vi "toCompiledXml.vi"(8 "error in (no error)":errorcluster, 11 "ScriptEvent in":refnum<class "ScriptEvent.lvclass">) -> (0 "error out":errorcluster, 2 "compiledXML":refnum<class "xmlNode.lvclass">, 3 "ScriptEvent out":refnum<class "ScriptEvent.lvclass">)   [LabVIEW 2011, in "Tools.lvlib" / "Scripting.lvlib" / "ScriptEvent.lvclass"]
uses:
  ScriptEvent.lvclass
  xmlNode/xmlNode.lvclass
  ScriptEvent.lvclass/ScriptEvent.ctl
  DatabaseHelpers/Database Objects/Channel/Channel.lvclass
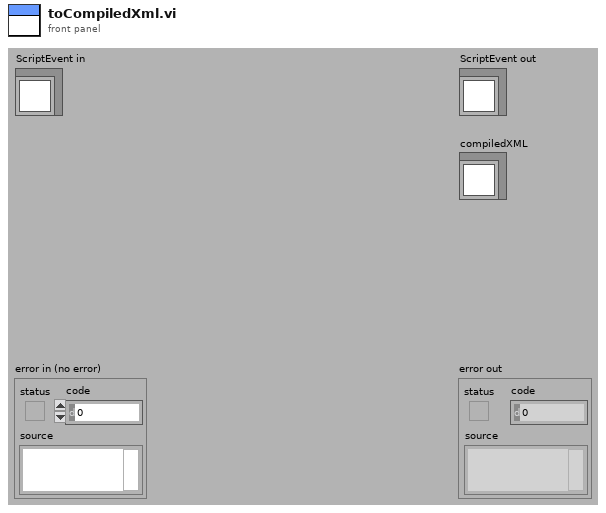
[diagram p1: front panel]
types:
  T1 = cluster{"attributeName":string, "channel_name":string}
  T2 = cluster{"attributeName":string, "channel_name":string}[]
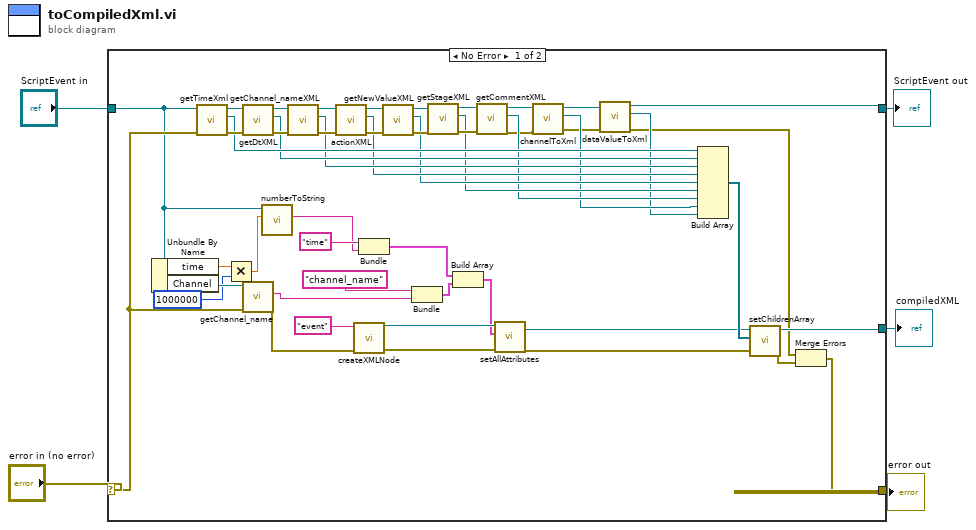
[diagram p0: block diagram]
diagram:
  n1 = case shown="No Error" "error in (no error)" {
    selector: "error in (no error)" -> [w40 w57]
    tunnel: [w29 w57] -> w2
    tunnel: [w7 w56] -> w4
    tunnel: "ScriptEvent in" -> [w14 w56]
    tunnel: [w31 _] -> w1
    frame No Error {
      n2 = Unbundle By Name(w14) -> ("time"=w18:dbl, "Channel"=w54:refnum<class "Channel.lvclass">)
      n3 = call "getTimeXml.vi"("error in (no error)"=w40, "ScriptEvent in"=w14) -> ("error out"=w52:errorcluster, "timeXML"=w39:refnum<class "xmlNode.lvclass">, "ScriptEvent out"=w46:refnum<class "ScriptEvent.lvclass">)  [unwired: 7 in]
      n4 = Multiply(x=w18, y=1000000) -> (x*y=w16:dbl)
      n5 = call "getDtXML.vi"("error in (no error)"=w52, "ScriptEvent in"=w46) -> ("error out"=w51:errorcluster, "dtXML"=w38:refnum<class "xmlNode.lvclass">, "ScriptEvent out"=w45:refnum<class "ScriptEvent.lvclass">)  [unwired: 7 in]
      n6 = call "getChannel_name.vi"("error in (no error)"=w40, "Channel.lvclass in"=w54) -> ("error out"=w53:errorcluster, "channel_name"=w26:string)  [unwired: 7 in, 1 out]
      n7 = call "numberToString.vi"("Numeric"=w16, "ScriptEvent in"=w14) -> ("String"=w15:string)  [unwired: 7 in, 2 out]
      n8 = call "getChannel_nameXML.vi"("error in (no error)"=w51, "ScriptEvent in"=w45) -> ("error out"=w50:errorcluster, "channel_nameXML"=w37:refnum<class "xmlNode.lvclass">, "ScriptEvent out"=w44:refnum<class "ScriptEvent.lvclass">)  [unwired: 7 in]
      n9 = call "actionXML.vi"("error in (no error)"=w50, "ScriptEvent in"=w44) -> ("error out"=w49:errorcluster, "actionXml"=w36:refnum<class "xmlNode.lvclass">, "ScriptEvent out"=w43:refnum<class "ScriptEvent.lvclass">)  [unwired: 7 in]
      n10 = call "createXMLNode.vi"("error in (no error)"=w53, "name"="event") -> ("error out"=w21:errorcluster, "xmlNode out"=w25:refnum<class "xmlNode.lvclass">)  [unwired: 8 in]
      n11 = Bundle("attributeName"="time", "String"=w15) -> (w24:cluster{"attributeName":string, "String":string})  [unwired: 1 in]
      n12 = call-dynamic "getNewValueXML.vi"("error in (no error)"=w49, "ScriptEvent in"=w43) -> ("error out"=w48:errorcluster, "newValueXML"=w35:refnum<class "xmlNode.lvclass">, "ScriptEvent out"=w42:refnum<class "ScriptEvent.lvclass">)  [unwired: 7 in]
      n13 = Bundle("attributeName"="channel_name", "channel_name"=w26) -> (w23:T1)  [unwired: 1 in]
      n14 = call "getStageXML.vi"("error in (no error)"=w48, "ScriptEvent in"=w42) -> ("error out"=w47:errorcluster, "stageXML"=w34:refnum<class "xmlNode.lvclass">, "ScriptEvent out"=w41:refnum<class "ScriptEvent.lvclass">)  [unwired: 7 in]
      n15 = Build Array(w24, w23) -> (w22:T2)
      n16 = call "getCommentXML.vi"("error in (no error)"=w47, "ScriptEvent in"=w41) -> ("error out"=w12:errorcluster, "commentXML"=w33:refnum<class "xmlNode.lvclass">, "ScriptEvent out"=w13:refnum<class "ScriptEvent.lvclass">)  [unwired: 7 in]
      n17 = call-dynamic "setAllAttributes.vi"("error in (no error)"=w21, "attributes"=w22, "xmlNode in"=w25) -> ("error out"=w20:errorcluster, "xmlNode out"=w19:refnum<class "xmlNode.lvclass">)  [unwired: 7 in]
      n18 = call "channelToXml.vi"("error in (no error)"=w12, "ScriptEvent in"=w13) -> ("error out"=w9:errorcluster, "xmlNode"=w11:refnum<class "xmlNode.lvclass">, "ScriptEvent out"=w10:refnum<class "ScriptEvent.lvclass">)  [unwired: 7 in]
      n19 = call-dynamic "dataValueToXml.vi"("error in (no error)"=w9, "ScriptEvent in"=w10) -> ("error out"=w6:errorcluster, "dataValueXml"=w8:refnum<class "xmlNode.lvclass">, "ScriptEvent out"=w7:refnum<class "ScriptEvent.lvclass">)  [unwired: 7 in]
      n20 = Build Array(w39, w38, w37, w36, w35, w34, w33, w11, w8) -> (w32:refnum<class "xmlNode.lvclass">[])
      n21 = call-dynamic "setChildrenArray.vi"("error in (no error)"=w20, "Children"=w32, "xmlNode.lvclass in"=w19) -> ("error out"=w30:errorcluster, "xmlNode.lvclass out"=w31:refnum<class "xmlNode.lvclass">)  [unwired: 7 in]
      n22 = Merge Errors(w6, w30) -> (w29:errorcluster)
    }
    frame Error {
    }
  }
  "error out" <- w2
  "ScriptEvent out" <- w4
  "compiledXML" <- w1
